vi "Find All Minima nD Prep.vi"(4 "Start":dbl[](array[numeric]) format="%.2f", 6 "X":string[](array[string]), 7 "F(X)":string, 8 "End":dbl[](array[numeric]) format="%.2f") -> (0 "error (general)":bool, 1 "Start":dbl[](array[numeric]) format="%.2f", 2 "time [msec]":u32, 3 "End":dbl[](array[numeric]) format="%.2f", 5 "specific error":bool)   [LabVIEW 2018, in "NI_Gmath.lvlib"]
uses:
  NI_Gmath.lvlib
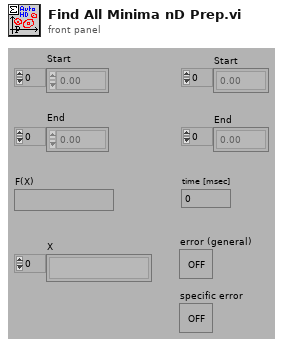
[diagram p1: front panel]
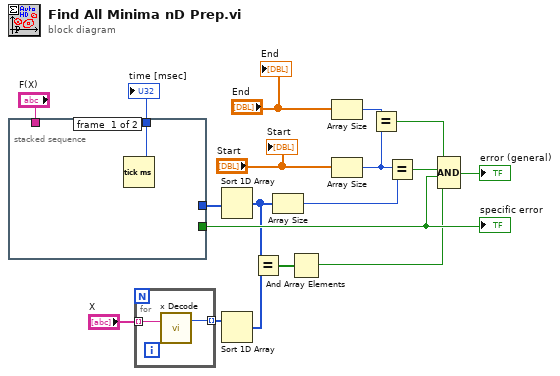
[diagram p0: block diagram]
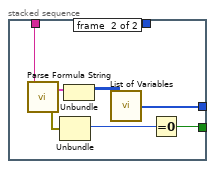
[diagram p2: hidden frame]
diagram:
  n1 = stacked-sequence {
    tunnel: [_ w26] -> w17
    tunnel: [w19 _] -> w4
    tunnel: [_ w25] -> w6
    tunnel: "F(X)" -> [_ w20]
    frame #0 {
      n2 = Tick Count (ms)() -> (millisecond timer value=w19:u32)
    }
    frame #1 {
      n3 = call "Parse Formula String.vi"("formula"=w20) -> ("error out"=w24:errorcluster, "Parsed Formula"=w23:cluster{"Table":i32[][], "Y Values":dbl[]})  [unwired: 1 in]
      n4 = Unbundle(w24) -> ("code"=w21:i32)  [unwired: 2 out]
      n5 = Unbundle(w23) -> ("Table"=w22:i32[][])  [unwired: 1 out]
      n6 = call "List of Variables.vi"("Table"=w22) -> ("List of variables"=w25:i32[])
      n7 = Equal To 0?(x=w21) -> (x = 0?=w26:bool)
    }
  }
  "specific error" <- w17
  "time [msec]" <- w4
  n8 = for {
    tunnel: "X" -> [w28] mode=indexing
    tunnel: [w27] -> w5 mode=indexing
    n9 = call "x Decode.vi"("x string"=w28) -> ("number"=w27:i32)  [unwired: 1 in, 1 out]
  }
  n10 = Sort 1D Array(array=w6) -> (sorted array=w8:i32[])
  n11 = Sort 1D Array(array=w5) -> (sorted array=w1:i32[])
  n12 = Equal?(x=w8, y=w1) -> (x = y?=w2:bool[])
  n13 = Array Size(array=w8) -> (size(s)=w13:i32)
  n14 = And Array Elements(Boolean array=w2) -> (logical AND=w3:bool)
  n15 = Array Size(array="End") -> (size(s)=w11:i32)
  n16 = Array Size(array="Start") -> (size(s)=w12:i32)
  n17 = Equal?(x=w11, y=w12) -> (x = y?=w14:bool)
  n18 = Equal?(x=w12, y=w13) -> (x = y?=w15:bool)
  n19 = Compound Arithmetic op=AND(w14, w15, w17, w3) -> (→"error (general)":bool)
  "End" <- "End"
  "Start" <- "Start"
